vi "Main.vi"() -> ()   [LabVIEW 2025]
doc: "本模板用于队列消息处理器设计模式。\n\n事件处理循环负责按用户界面操作生成对应的消息。\n\n消息处理循环负责对事件处理循环或其他消息生成的消息进行处理。消息内容为字符串值，因此很容易将新消息添加至“消息处理”循环的“消息分支”条件结构。每个消息簇还可选择性地为消息数据提供一个变体，变体数据可以转换为消息数据所需要的任意类型。"
uses:
  controls/UI Data.ctl
  support/Message Queue/Enqueue Message (Single).vi
  <vilib>/Instr/_visa.llb/VISA Configure Serial Port (Instr).vi
  <vilib>/Utility/error.llb/Error Cluster From Error Code.vi
  <vilib>/ErrorRing/Error Ring.xnode
  support/Message Queue/Message Queue.lvlib
  support/User Event - Stop/User Event - Stop.lvlib
panel:
  in  "土壤湿度":dbl(slide) scale=0.0..100.0
  in  "关灯":bool
  out "数据":string
  in  "退出":bool
  out "正常运行":bool
  in  "Vertical Pause Button":bool
  in  "Vertical Start Button":bool
  in  "System Save Data Button":bool
  in  "停止":bool
  in  "开灯":bool
  out "输出":string
  in  "输入":string
  in  "采集":bool
  in  "串口":refnum<visa-resource-name>
  in  "停止位":u16
  in  "数据比特":u16
  in  "奇偶校验":u16
  in  "波特率":u16
  out "光照":dbl(knob) scale=0.0..100000.0
  out "光照报警":bool
  out "湿度报警":bool
  out "温度报警":bool
  in  "湿度":dbl(slide) scale=0.0..100.0
  out "环境数据实时趋势曲线":cluster{dbl, dbl}[](graph)
  out "温度":i16(slide) scale=0.0..60.0
  out "显示<替换此项>":string
  in  "执行其他操作<替换此项>":bool
  in  "执行某操作<替换此项>":bool
  # "环境数据采集"
  # "控制"
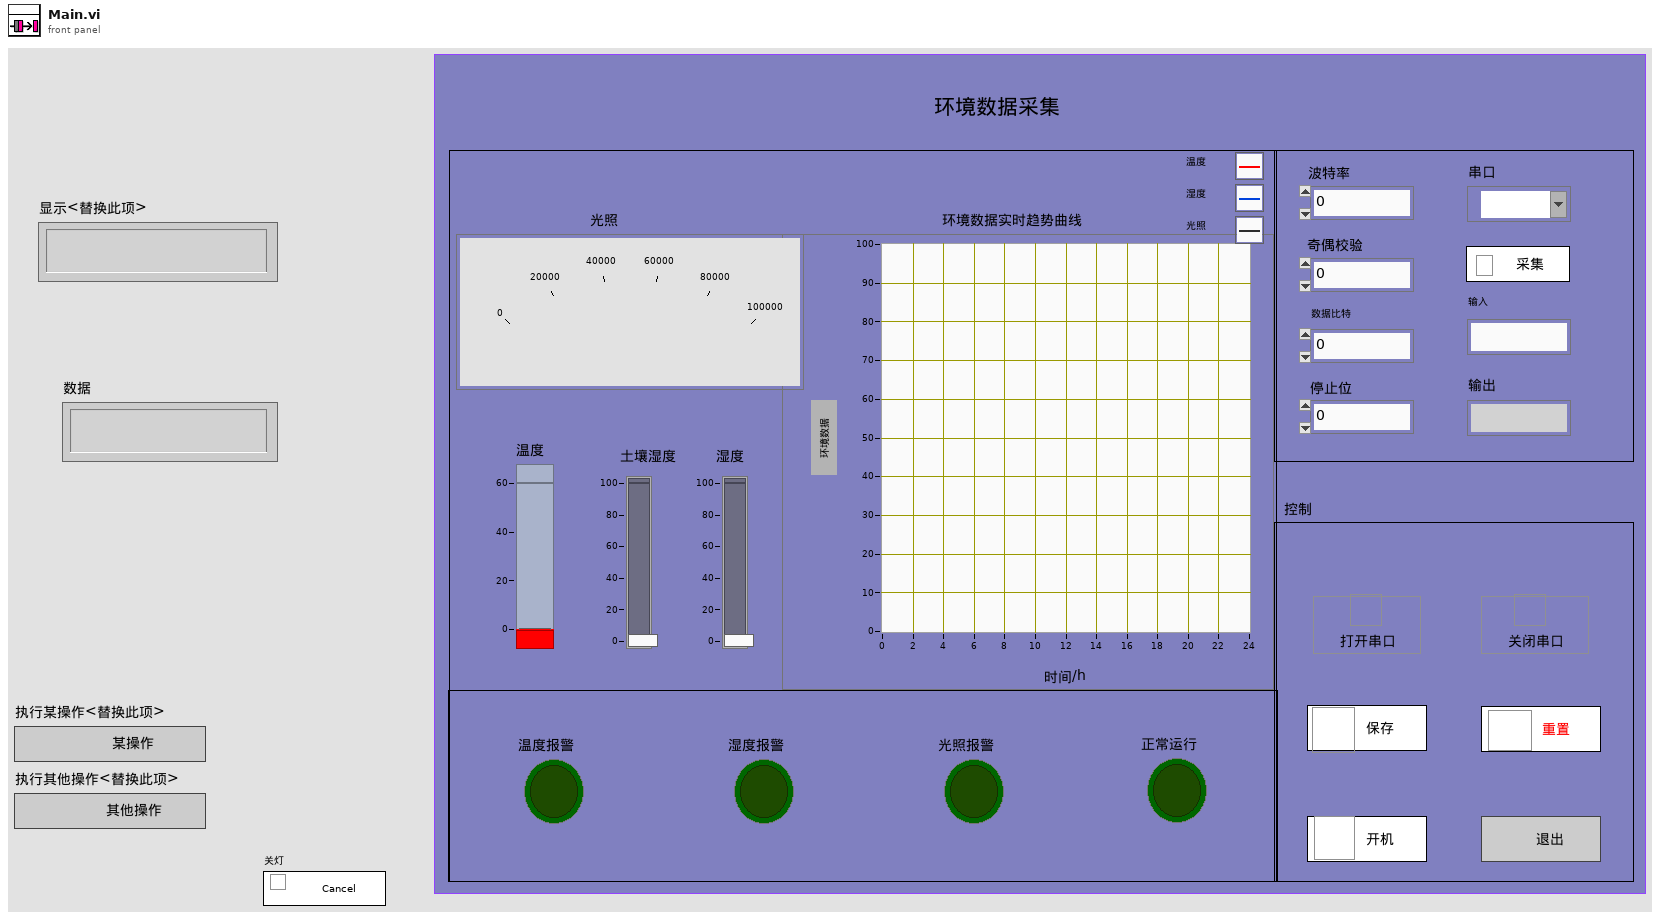
[diagram p1: front panel]
types:
  T1 = typedef "UI Data.ctl" = cluster{"布尔<替换此项>":bool, "字符串<替换此项>":string, "数值<替换此项>":dbl, "执行某操作引用":refnum<vi>, "执行其他操作引用":refnum<vi>, "数据显示引用":refnum<vi>, "退出按钮引用":refnum<vi>}
  T2 = typedef "Message Queue.lvlib/All Message Queues.ctl" = cluster{"UI":refnum<queue>, "数据":refnum<queue>, "采集":refnum<queue>, "控制":refnum<queue>}
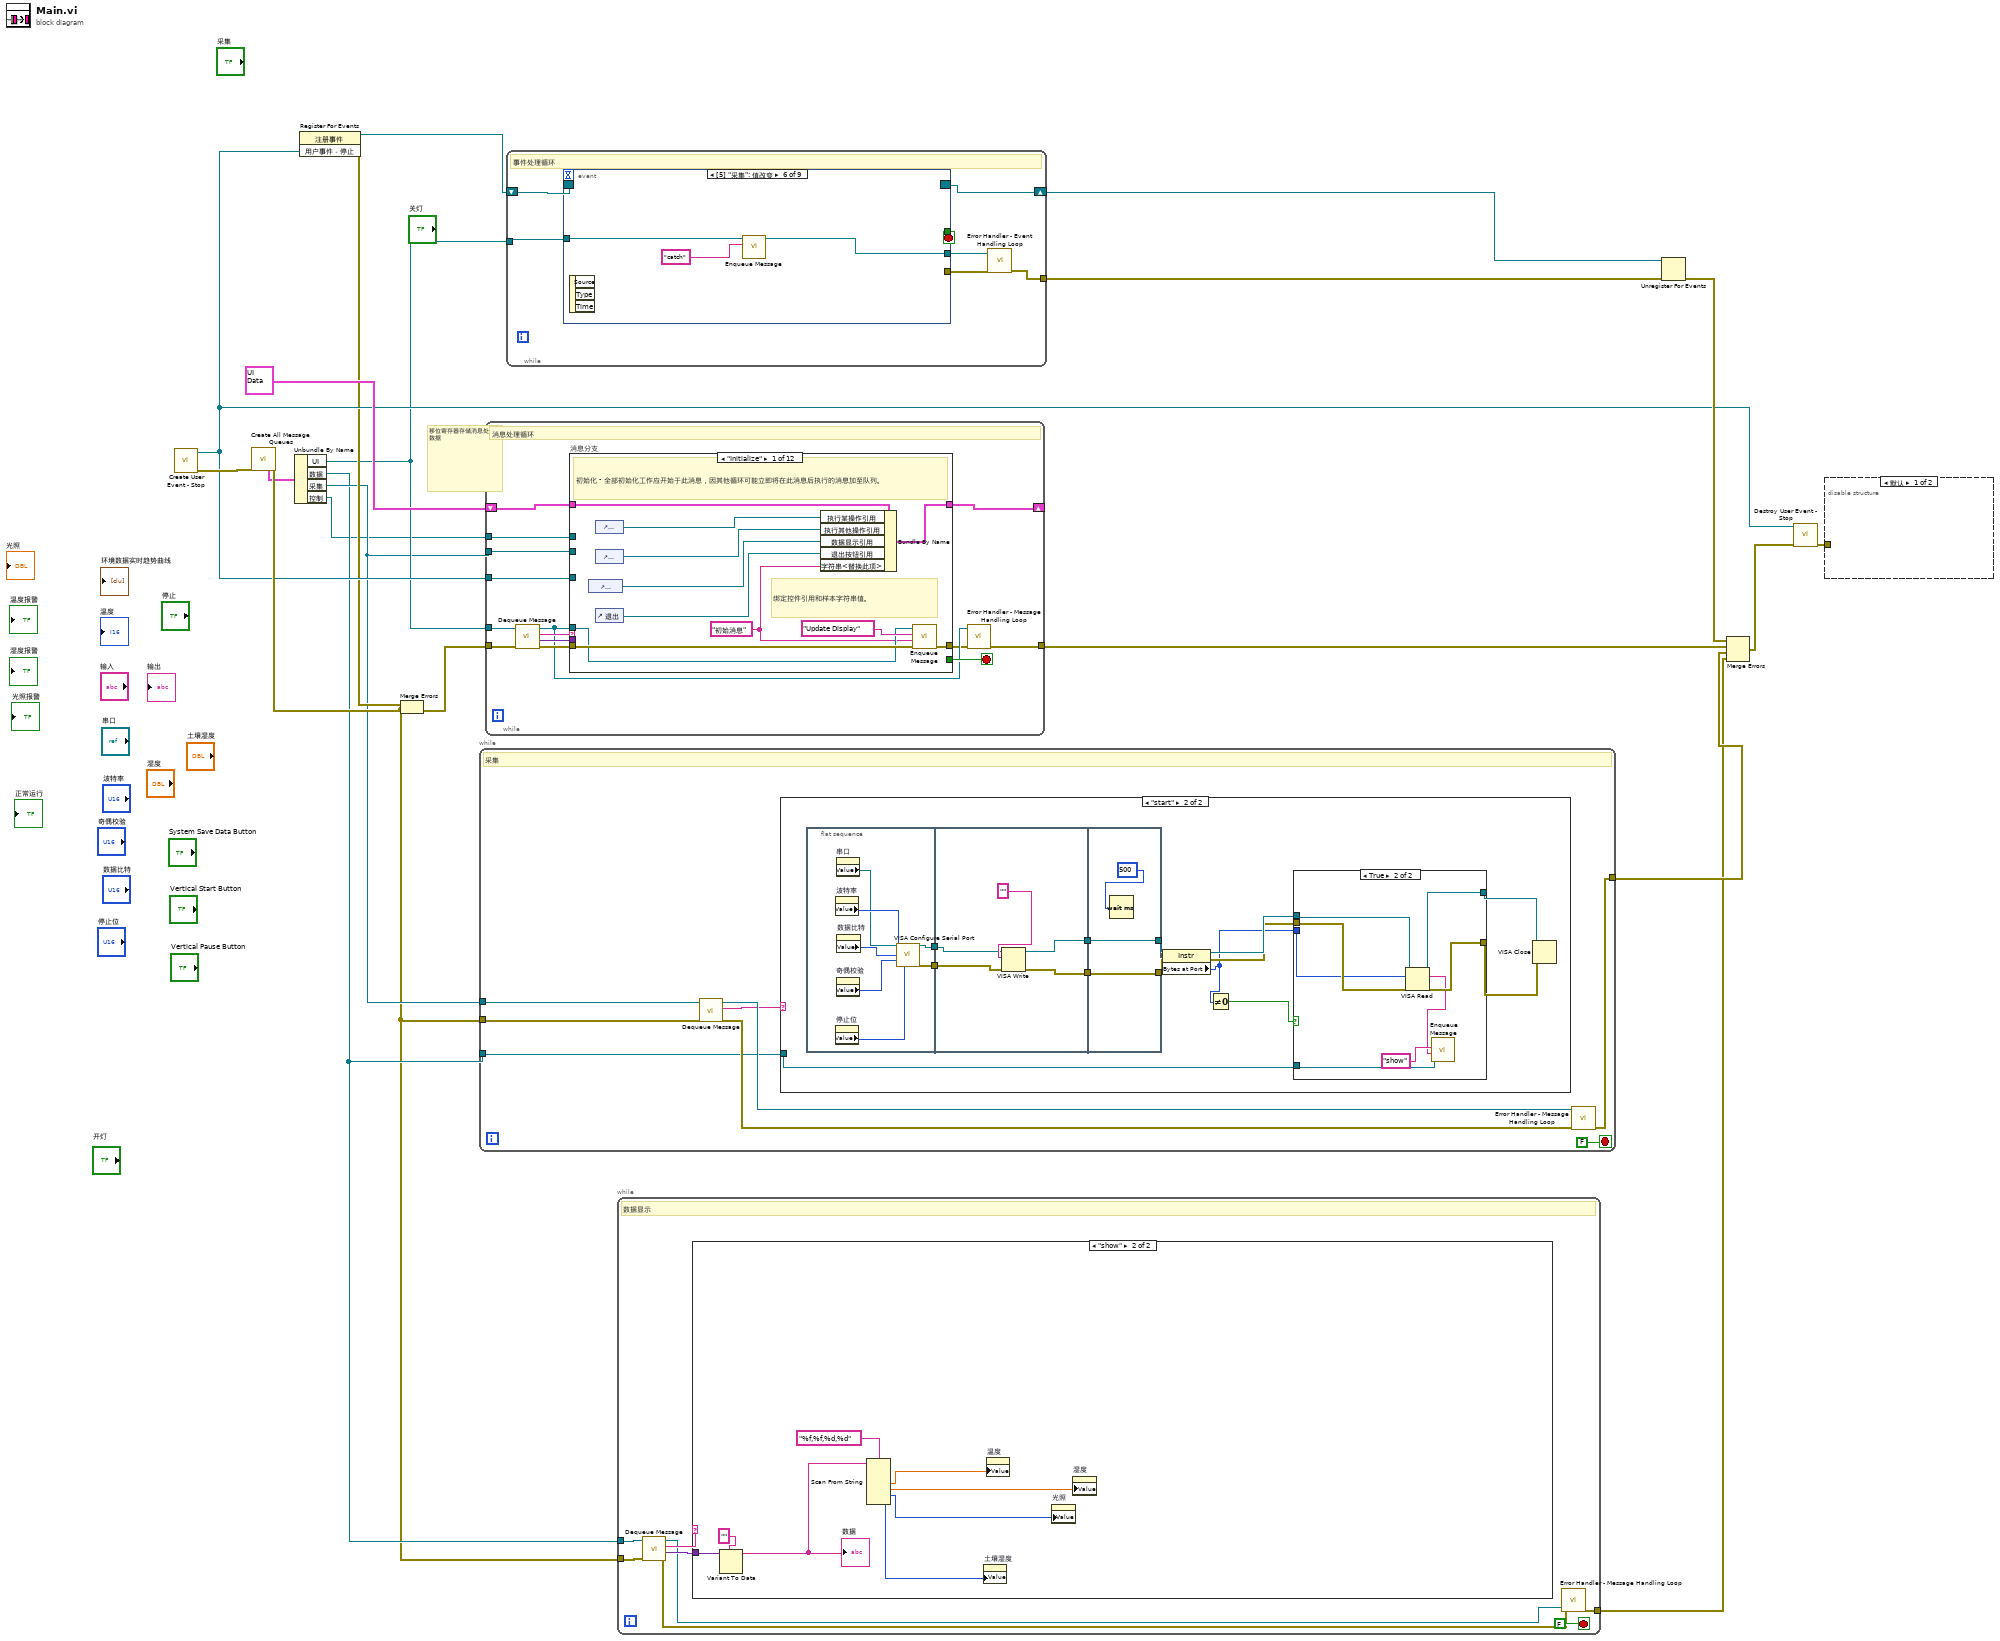
[diagram p0: block diagram]
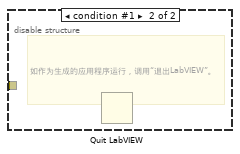
[diagram p5: hidden frame]
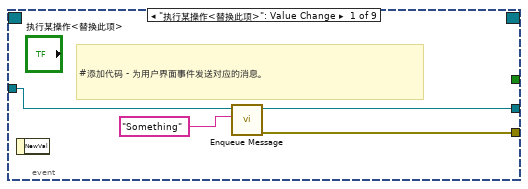
[diagram p6: hidden frame]
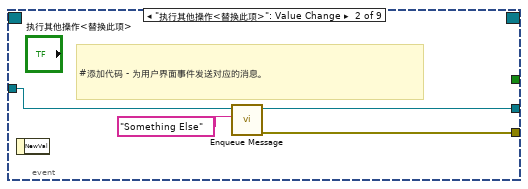
[diagram p7: hidden frame]
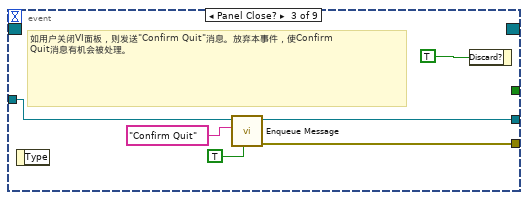
[diagram p8: hidden frame]
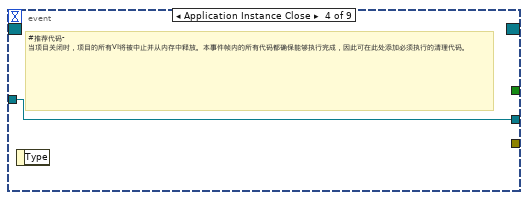
[diagram p9: hidden frame]
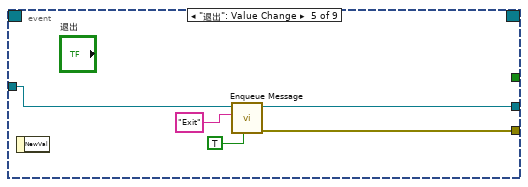
[diagram p10: hidden frame]
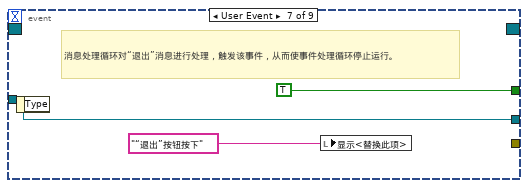
[diagram p11: hidden frame]
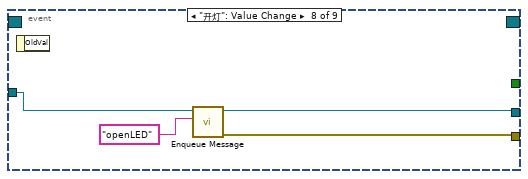
[diagram p12: hidden frame]
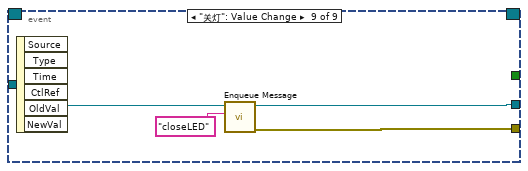
[diagram p13: hidden frame]
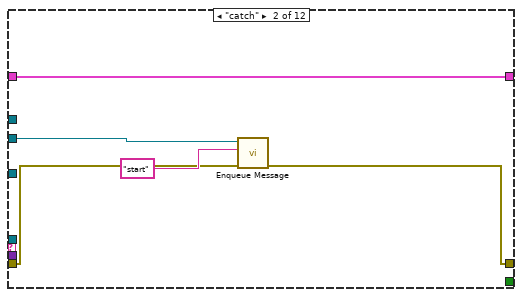
[diagram p14: hidden frame]
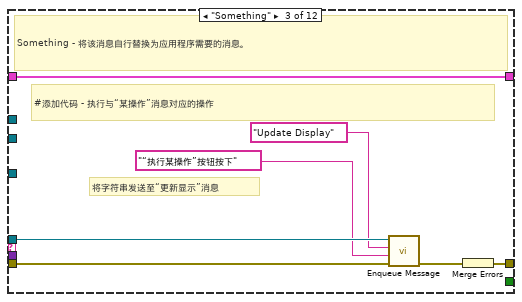
[diagram p15: hidden frame]
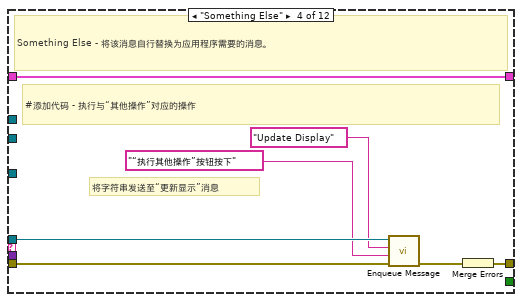
[diagram p16: hidden frame]
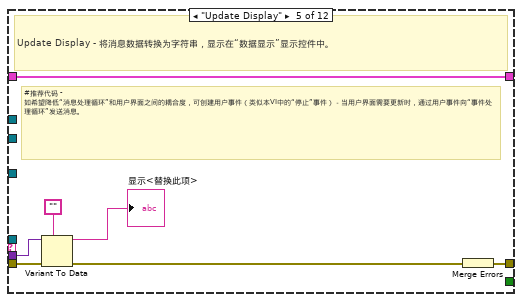
[diagram p17: hidden frame]
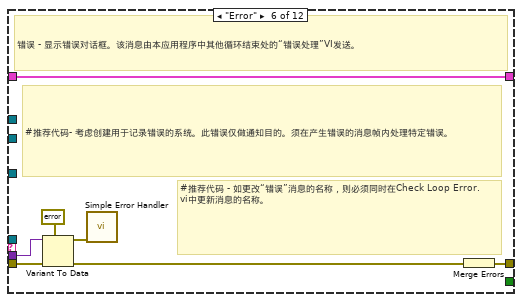
[diagram p18: hidden frame]
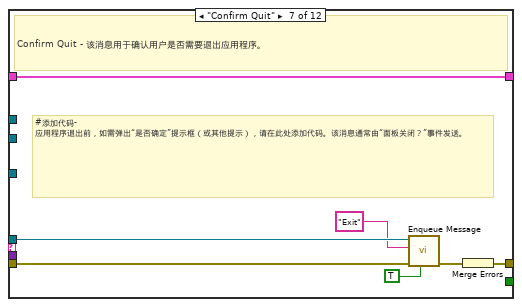
[diagram p19: hidden frame]
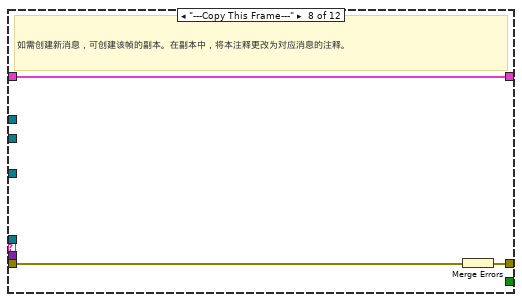
[diagram p20: hidden frame]
diagram:
  # "移位寄存器存储消息处理器的数据"
  n1 = call "Create User Event - Stop.vi"() -> ("error out"=w17:cluster{"状态":bool, "代码":i32, "源":string}, "用户事件－停止"=w9:refnum<user-event>)  [unwired: 10 in]
  n2 = call "Create All Message Queues.vi"("error in (no error)"=w17) -> ("error out"=w20:cluster{"状态":bool, "代码":i32, "源":string}, "消息队列输出"=w19:T2)  [unwired: 9 in]
  n3 = Unbundle By Name(w19) -> ("UI"=w7:refnum<queue>, "数据"=w4:refnum<queue>, "采集"=w6:refnum<queue>, "控制"=w1:refnum<queue>)
  n4 = register-events(w9) -> (reference out=w10:refnum<event-registration>, error out=w8:errorcluster)  [unwired: 2 in]
  n5 = Merge Errors(w8, w20) -> (w3:errorcluster)
  n6 = while {
    tunnel: w6 -> [w27]
    tunnel: w3 -> [w26]
    tunnel: [w25] -> w5
    tunnel: w4 -> [w21]
    stop <- FALSE stop-if-true
    # "采集"
    n7 = call "Dequeue Message.vi"("error in (no error)"=w26, "消息队列"=w27) -> ("error out"=w24:cluster{"状态":bool, "代码":i32, "源":string}, "消息"=w22:string, "消息队列副本"=w23:refnum<queue>)  [unwired: 6 in, 1 out]
    n8 = case shown="\"start\"" w22 {
      tunnel: w21 -> [_ w36]
      frame "False", Default {
      }
      frame "start" {
        n9 = flat-sequence {
          tunnel: [w43] -> w35
          tunnel: [w42] -> w34
          tunnel: w35 -> [w51]
          tunnel: w34 -> [w53]
          tunnel: [w50] -> w31
          tunnel: [w49] -> w30
          tunnel: [w55] -> w32
          tunnel: [w56] -> w33
          tunnel: w31 -> [w56]
          tunnel: w30 -> [w55]
          frame #0 {
            n10 = property on="波特率" class="DigNum (严格)"() -> ("Value"=w48:u16)  [unwired: 2 in, 2 out]
            n11 = property on="停止位" class="DigNum (严格)"() -> ("Value"=w47:u16)  [unwired: 2 in, 2 out]
            n12 = property on="串口" class="VISAName"() -> ("Value"=w44:refnum<visa-resource-name>)  [unwired: 2 in, 2 out]
            n13 = property on="奇偶校验" class="DigNum (严格)"() -> ("Value"=w45:u16)  [unwired: 2 in, 2 out]
            n14 = property on="数据比特" class="DigNum (严格)"() -> ("Value"=w46:u16)  [unwired: 2 in, 2 out]
            n15 = call-poly "VISA Configure Serial Port"("VISA resource name"=w44, "baud rate (9600)"=w48, "data bits (8)"=w46, "parity (0:none)"=w45, "stop bits (10: 1 bit)"=w47) -> ("VISA resource name out"=w43:refnum<visa-resource-name>, "error out"=w42:errorcluster)  [unwired: 9 in]
          }
          frame #1 {
            n16 = VISA Write(VISA resource name=w51, write buffer="", error in (no error)=w53) -> (VISA resource name out=w49:refnum<visa-resource-name>, error out=w50:errorcluster)  [unwired: 1 out]
          }
          frame #2 {
            n17 = Wait (ms)(milliseconds to wait=500) -> ()  [unwired: 1 out]
          }
        }
        n18 = property class="Instr"(reference=w32, error in=w33) -> (reference out=w41:refnum<visa-resource-name>, error out=w39:errorcluster, "Bytes at Port"=w37:u32)
        n19 = Not Equal To 0?(x=w37) -> (x != 0?=w29:bool)
        n20 = case shown="True" w29 {
          tunnel: w41 -> [w58 w66]
          tunnel: [w58 w60] -> w40
          tunnel: w39 -> [w57 w65]
          tunnel: [w57 w64] -> w38
          tunnel: w37 -> [_ w63]
          tunnel: w36 -> [_ w61]
          frame False {
          }
          frame True {
            n21 = VISA Read(VISA resource name=w66, byte count=w63, error in (no error)=w65) -> (VISA resource name out=w60:refnum<visa-resource-name>, read buffer=w59:string, error out=w64:errorcluster)  [unwired: 1 out]
            n22 = call-poly "Enqueue Message.vi"("消息数据"=w59, "消息"="show", "消息队列"=w61) -> ()  [unwired: 7 in, 2 out]
          }
        }
        n23 = VISA Close(VISA resource name=w40, error in (no error)=w38) -> ()  [unwired: 1 out]
      }
    }
    n24 = call "Error Handler - Message Handling Loop.vi"("error in (no error)"=w24, "消息队列"=w23) -> ("错误输入副本"=w25:cluster{"状态":bool, "代码":i32, "源":string})  [unwired: 8 in, 1 out]
  }
  n25 = while {
    tunnel: w7 -> [w72]
    shift-right: [w79] -> _
    shift-left: T1 {"布尔<替换此项>"=FALSE, "字符串<替换此项>"="", "数值<替换此项>"=0.0, "执行某操作引用"=refnum, "执行其他操作引用"=refnum, "数据显示引用"=refnum, "退出按钮引用"=refnum} ("Data Cluster") -> [w80]
    tunnel: w9 -> [w77]
    tunnel: w3 -> [w76]
    tunnel: [w70] -> w18
    tunnel: w6 -> [w68]
    tunnel: w1 -> [w67]
    stop <- w78 stop-if-true
    # "消息处理循环"
    n26 = call "Dequeue Message.vi"("error in (no error)"=w76, "消息队列"=w72) -> ("error out"=w75:cluster{"状态":bool, "代码":i32, "源":string}, "消息数据"=w73:variant, "消息"=w74:string, "消息队列副本"=w71:refnum<queue>)  [unwired: 6 in]
    n27 = case "消息分支" shown="\"Initialize\"" w74 {
      selector: w74 -> [_ _ _ _ _ _ _ _ _ _ _ w155]
      tunnel: w71 -> [w82 _ w99 w106 _ _ w127 _ w145 _ _ _]
      tunnel: w75 -> [w90 w93 w101 w108 w115 w124 w131 w134 w138 w147 w154 _]
      tunnel: [w91 w92 w102 w109 w116 w118 w129 w132 w141 w146 w154 w156] -> w69
      tunnel: w80 -> [w89 w96 w103 w110 w117 w123 w130 w133 w144 w150 w153 w157]
      tunnel: [w88 w96 w103 w110 w117 w123 w130 w133 w144 w150 w153 w157] -> w79
      tunnel: [_ _ _ _ _ _ _ _ TRUE _ _ _] -> w78
      tunnel: w73 -> [_ _ _ _ w114 w122 _ _ w135 _ _ _]
      tunnel: w77 -> [_ _ _ _ _ _ _ _ w140 _ _ _]
      tunnel: w68 -> [_ w95 _ _ _ _ _ _ _ _ _ _]
      tunnel: w67 -> [_ _ _ _ _ _ _ _ _ w148 w151 _]
      frame "Initialize" {
        w81 = "初始消息" ("Initial Message")
        # "绑定控件引用和样本字符串值。"
        # "初始化 - 全部初始化工作应开始于此消息，因其他循环可能立即将在此消息后执行的消息加至队列。"
        n28 = control-ref of="显示<替换此项>"() -> (w85:refnum<vi>)
        n29 = control-ref of="执行某操作<替换此项>"() -> (w87:refnum<vi>)
        n30 = control-ref of="执行其他操作<替换此项>"() -> (w86:refnum<vi>)
        n31 = control-ref of="退出"() -> (w84:refnum<vi>)
        n32 = Bundle By Name(cluster=w89, "执行某操作引用"=w87, "执行其他操作引用"=w86, "数据显示引用"=w85, "退出按钮引用"=w84, "字符串<替换此项>"=w81) -> (w88:T1)
        n33 = call-poly "Enqueue Message.vi"("error in (no error)"=w90, "消息数据"=w81, "消息"="Update Display" ("Message"), "消息队列"=w82) -> ("error out"=w91:cluster{"状态":bool, "代码":i32, "源":string})  [unwired: 6 in, 1 out]
      }
      frame "catch" {
        n34 = call-poly "Enqueue Message.vi"("error in (no error)"=w93, "消息"="start", "消息队列"=w95) -> ("error out"=w92:cluster{"状态":bool, "代码":i32, "源":string})  [unwired: 7 in, 1 out]
      }
      frame "Something" {
        # "将字符串发送至“更新显示”消息"
        # "#添加代码 - 执行与“某操作”消息对应的操作"
        # "Something - 将该消息自行替换为应用程序需要的消息。"
        n35 = call-poly "Enqueue Message.vi"("error in (no error)"=w101, "消息数据"="“执行某操作”按钮按下" ("\"Do Something\" button pressed"), "消息"="Update Display" ("Message"), "消息队列"=w99) -> ("error out"=w100:cluster{"状态":bool, "代码":i32, "源":string})  [unwired: 6 in, 1 out]
        n36 = Merge Errors(w100) -> (w102:errorcluster)
      }
      frame "Something Else" {
        # "将字符串发送至“更新显示”消息"
        # "#添加代码 - 执行与“其他操作”对应的操作"
        # "Something Else - 将该消息自行替换为应用程序需要的消息。"
        n37 = call-poly "Enqueue Message.vi"("error in (no error)"=w108, "消息数据"="“执行其他操作”按钮按下" ("\"Do Something Else\" button pressed"), "消息"="Update Display" ("Message"), "消息队列"=w106) -> ("error out"=w107:cluster{"状态":bool, "代码":i32, "源":string})  [unwired: 6 in, 1 out]
        n38 = Merge Errors(w107) -> (w109:errorcluster)
      }
      frame "Update Display" {
        # "#推荐代码 - 如希望降低“消息处理循环”和用户界面之间的耦合度，可创建用户事件（类似本VI中的“停止”事件）－当用户界面需要更新时，通过用户事件向“事件处理循环”发送消息。"
        # "Update Display - 将消息数据转换为字符串，显示在“数据显示”显示控件中。"
        n39 = Variant To Data(error in=w115, type="", Variant=w114) -> (data=→"显示<替换此项>":string, error out=w112:errorcluster)
        n40 = Merge Errors(w112) -> (w116:errorcluster)
      }
      frame "Error" {
        # "#推荐代码 - 如更改“错误”消息的名称，则必须同时在Check Loop Error.vi中更新消息的名称。"
        # "#推荐代码- 考虑创建用于记录错误的系统。此错误仅做通知目的。须在产生错误的消息帧内处理特定错误。"
        # "错误 - 显示错误对话框。该消息由本应用程序中其他循环结束处的“错误处理”VI发送。"
        n41 = Variant To Data(error in=w124, type=errorcluster {"status"=FALSE, "code"=0, "source"=""} ("error constant"), Variant=w122) -> (data=w120:errorcluster, error out=w119:errorcluster)
        n42 = call <vilib>:"Simple Error Handler.vi"("error in (no error)"=w120) -> ()  [unwired: 4 in, 5 out]
        n43 = Merge Errors(w119) -> (w118:errorcluster)
      }
      frame "Confirm Quit" {
        # "#添加代码- 应用程序退出前，如需弹出“是否确定”提示框（或其他提示），请在此处添加代码。该消息通常由“面板关闭？”事件发送。"
        # "Confirm Quit - 该消息用于确认用户是否需要退出应用程序。"
        n44 = call-poly "Enqueue Message.vi"("优先消息？ (F)"=TRUE ("Priority Message? (F)"), "error in (no error)"=w131, "消息"="Exit" ("Message"), "消息队列"=w127) -> ("error out"=w128:cluster{"状态":bool, "代码":i32, "源":string})  [unwired: 6 in, 1 out]
        n45 = Merge Errors(w128) -> (w129:errorcluster)
      }
      frame "---Copy This Frame---" {
        # "如需创建新消息，可创建该帧的副本。在副本中，将本注释更改为对应消息的注释。"
        n46 = Merge Errors(w134) -> (w132:errorcluster)
      }
      frame "Exit" {
        # "停止VI"
        # "释放消息队列引用"
        # "#添加代码 - 此处按需要添加清理代码注意，如果'退出' 作为错误结果被调用，则将显示错误对话框。为“退出”条件添加自定义错误处理。"
        # "Exit - 退出应用程序。"
        n47 = Variant To Data(type=errorcluster {"status"=FALSE, "code"=0, "source"=""} ("error constant"), Variant=w135) -> (data=w136:errorcluster)  [unwired: 1 in, 1 out]
        n48 = call <vilib>:"Simple Error Handler.vi"("error in (no error)"=w136) -> ()  [unwired: 4 in, 5 out]
        n49 = call "Fire User Event - Stop.vi"("用户事件－停止"=w140) -> ("error out"=w139:cluster{"状态":bool, "代码":i32, "源":string})  [unwired: 10 in]
        n50 = Release Queue(queue=w145, error in (no error)=w138) -> (error out=w142:errorcluster)  [unwired: 1 in, 2 out]
        n51 = Merge Errors(w139, w142) -> (w141:errorcluster)
      }
      frame "openLED" {
        n52 = call-poly "Enqueue Message.vi"("error in (no error)"=w147, "消息"="OPENLED", "消息队列"=w148) -> ("error out"=w146:cluster{"状态":bool, "代码":i32, "源":string})  [unwired: 7 in, 1 out]
      }
      frame "closeLED" {
        n53 = call-poly "Enqueue Message.vi"("消息"="CLOSELED", "消息队列"=w151) -> ()  [unwired: 8 in, 2 out]
      }
      frame Default {
        # "如得到的消息未经任何分支定义，则运行“默认”分支。输出程序错误。"
        n54 = xnode ("Error Ring")("parameter 0"=w155) -> ("error out"=w156:errorcluster)
      }
    }
    n55 = call "Error Handler - Message Handling Loop.vi"("error in (no error)"=w69, "消息队列"=w71) -> ("错误输入副本"=w70:cluster{"状态":bool, "代码":i32, "源":string})  [unwired: 8 in, 1 out]
  }
  n56 = while {
    shift-right: [w170] -> w14
    shift-left: w10 -> [w171]
    tunnel: [w166] -> w11
    tunnel: w7 -> [w165]
    stop <- w168 stop-if-true
    # "事件处理循环"
    n57 = event shown="[5] \"采集\": 值改变" {
      selector: w171 -> [_ _ _ _ _ _ _ _ _]
      dyn-events: [_ _ _ _ _ _ _ _ _] -> w170
      timeout: _ -> [_ _ _ _ _ _ _ _ _]
      tunnel: [_ _ _ _ _ _ TRUE ("Discard?") _ _] -> w168
      tunnel: [w173 w177 w184 _ w191 _ _ w201 w205] -> w169
      tunnel: [w175 w179 w183 w186 w190 w193 w195 w198 w202] -> w167
      tunnel: w165 -> [w172 w176 w180 w186 w187 w194 w195 w199 w203]
      event "执行某操作<替换此项>": Value Change {
        # "#添加代码 - 为用户界面事件发送对应的消息。"
        n58 = event-data() -> ()  [unwired: 1 in, 1 out]
        n59 = call-poly "Enqueue Message.vi"("消息"="Something" ("Message"), "消息队列"=w172) -> ("error out"=w173:cluster{"状态":bool, "代码":i32, "源":string}, "消息队列副本"=w175:refnum<queue>)  [unwired: 8 in]
      }
      event "执行其他操作<替换此项>": Value Change {
        # "#添加代码 - 为用户界面事件发送对应的消息。"
        n60 = event-data() -> ()  [unwired: 1 in, 1 out]
        n61 = call-poly "Enqueue Message.vi"("消息"="Something Else" ("Message"), "消息队列"=w176) -> ("error out"=w177:cluster{"状态":bool, "代码":i32, "源":string}, "消息队列副本"=w179:refnum<queue>)  [unwired: 8 in]
      }
      event Panel Close? {
        # "如用户关闭VI面板，则发送\"Confirm Quit\"消息。放弃本事件，使Confirm Quit消息有机会被处理。"
        n62 = event-data() -> ()  [unwired: 1 in, 1 out]
        n63 = call-poly "Enqueue Message.vi"("优先消息？ (F)"=TRUE ("Priority Message? (F)"), "消息"="Confirm Quit" ("Message"), "消息队列"=w180) -> ("error out"=w184:cluster{"状态":bool, "代码":i32, "源":string}, "消息队列副本"=w183:refnum<queue>)  [unwired: 7 in]
        n64 = event-data ("Event Filter Node")("Discard?"=TRUE) -> ()  [unwired: 1 in, 1 out]
      }
      event Application Instance Close {
        # "#推荐代码- 当项目关闭时，项目的所有VI将被中止并从内存中释放。本事件帧内的所有代码都确保能够执行完成，因此可在此处添加必须执行的清理代码。"
        n65 = event-data() -> ()  [unwired: 1 in, 1 out]
      }
      event "退出": Value Change {
        n66 = event-data() -> ()  [unwired: 1 in, 1 out]
        n67 = call-poly "Enqueue Message.vi"("优先消息？ (F)"=TRUE ("Priority Message? (F)"), "消息"="Exit" ("Message"), "消息队列"=w187) -> ("error out"=w191:cluster{"状态":bool, "代码":i32, "源":string}, "消息队列副本"=w190:refnum<queue>)  [unwired: 7 in]
      }
      event "采集": Value Change {
        n68 = event-data() -> ()  [unwired: 1 in, 3 out]
        n69 = call-poly "Enqueue Message.vi"("消息"="catch", "消息队列"=w194) -> ("消息队列副本"=w193:refnum<queue>)  [unwired: 8 in, 1 out]
      }
      event User Event {
        # "消息处理循环对“退出”消息进行处理，触发该事件，从而使事件处理循环停止运行。"
        n70 = event-data() -> ()  [unwired: 1 in, 1 out]
        n71 = local write "显示<替换此项>"("“退出”按钮按下" ("VI Stopped")) -> ()
      }
      event "开灯": Value Change {
        n72 = event-data() -> ()  [unwired: 1 in, 1 out]
        n73 = call-poly "Enqueue Message.vi"("消息"="openLED", "消息队列"=w199) -> ("error out"=w201:cluster{"状态":bool, "代码":i32, "源":string}, "消息队列副本"=w198:refnum<queue>)  [unwired: 8 in]
      }
      event "关灯": Value Change {
        n74 = event-data() -> ()  [unwired: 1 in, 6 out]
        n75 = call-poly "Enqueue Message.vi"("消息"="closeLED", "消息队列"=w203) -> ("error out"=w205:cluster{"状态":bool, "代码":i32, "源":string}, "消息队列副本"=w202:refnum<queue>)  [unwired: 8 in]
      }
    }
    n76 = call "Error Handler - Event Handling Loop.vi"("error in (no error)"=w169, "消息队列"=w167) -> ("错误输入副本"=w166:cluster{"状态":bool, "代码":i32, "源":string})  [unwired: 8 in, 1 out]
  }
  n77 = while {
    tunnel: w4 -> [w212]
    tunnel: w3 -> [w209]
    tunnel: [w206] -> w2
    stop <- FALSE stop-if-true
    # "数据显示"
    n78 = call "Dequeue Message.vi"("error in (no error)"=w209, "消息队列"=w212) -> ("error out"=w208:cluster{"状态":bool, "代码":i32, "源":string}, "消息数据"=w210:variant, "消息"=w211:string, "消息队列副本"=w207:refnum<queue>)  [unwired: 6 in]
    n79 = case shown="\"show\"" w211 {
      tunnel: w210 -> [_ w221]
      frame "False", Default {
      }
      frame "show" {
        n80 = Variant To Data(type="", Variant=w221) -> (data=w219:string)  [unwired: 1 in, 1 out]
        "数据" <- w219
        n81 = Scan From String(format string="%f,%f,%d,%d" ("格式字符串"), input string=w219) -> (output 1=w217:dbl, output 2=w216:dbl, output 3=w215:i32, output 4=w214:i32)  [unwired: 6 in, 3 out]
        n82 = property on="土壤湿度" class="Slide (严格)"("Value"=w214) -> ()  [unwired: 2 in, 2 out]
        n83 = property on="温度" class="Slide (严格)"("Value"=w217) -> ()  [unwired: 2 in, 2 out]
        n84 = property on="光照" class="Knob (严格)"("Value"=w215) -> ()  [unwired: 2 in, 2 out]
        n85 = property on="湿度" class="Slide (严格)"("Value"=w216) -> ()  [unwired: 2 in, 2 out]
      }
    }
    n86 = call "Error Handler - Message Handling Loop.vi"("error in (no error)"=w208, "消息队列"=w207) -> ("错误输入副本"=w206:cluster{"状态":bool, "代码":i32, "源":string})  [unwired: 8 in, 1 out]
  }
  n87 = Unregister For Events(event registration refnum=w14, error in=w11) -> (error out=w15:errorcluster)
  n88 = Merge Errors(w15, w18, w5, w2) -> (w16:errorcluster)
  n89 = call "Destroy User Event - Stop.vi"("error in (no error)"=w16, "用户事件－停止"=w9) -> ("error out"=w12:cluster{"状态":bool, "代码":i32, "源":string})  [unwired: 9 in]
  n90 = disable-structure "Conditional Disable Structure" shown="默认" {
    disable-tunnel: w12 -> [_ _]
    frame condition #0 (active) {
    }
    frame condition #1 {
      # "如作为生成的应用程序运行，调用“退出LabVIEW”。"
      n91 = Quit LabVIEW() -> ()  [unwired: 1 in]
    }
  }
